vi "Query Relative Amplitude Limit Auto Enabled.vi"(8 "error in (no error)":errorcluster {"code" format="%.0x"}, 9 "RetValBufferSize":i32=2048, 11 "instrument handle":refnum<k15>) -> (0 "error out":errorcluster {"code" format="%.0x"}, 1 "RetValActualSize":i32, 2 "RetVal":u16[](array[numeric]), 3 "instrument handle out":refnum<k15>)   [LabVIEW 2021, in "Keysight XSAnVMA.lvlib"]
doc: "Gets state of relative power level limit at the stop frequency for the selected offset."
uses:
  <instrlib>/Keysight XSAnVMA/Keysight XSAnVMA.lvlib
  KtXSAnVMA_64.dll
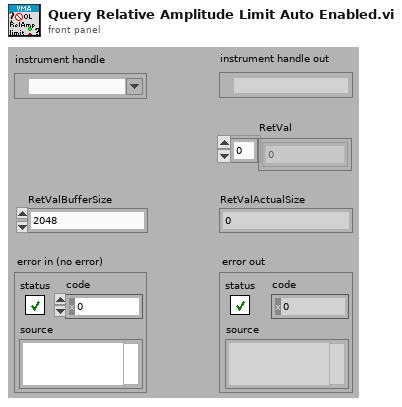
[diagram p1: front panel]
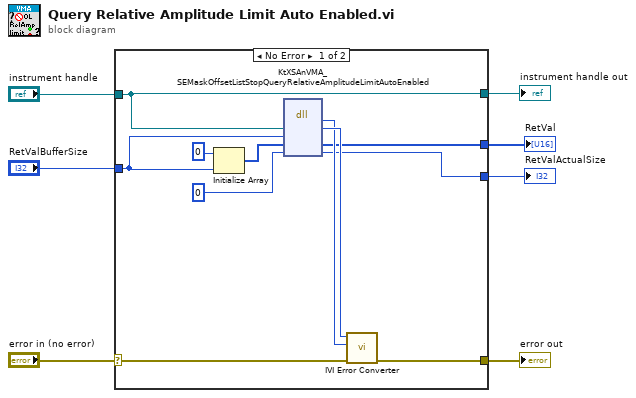
[diagram p0: block diagram]
diagram:
  n1 = case shown="No Error" "error in (no error)" {
    selector: "error in (no error)" -> [w16 w20]
    tunnel: [w15 w20] -> w7
    tunnel: "instrument handle" -> [w9 w19]
    tunnel: "RetValBufferSize" -> [w8 _]
    tunnel: [w12 _] -> w3
    tunnel: [w10 _] -> w2
    tunnel: [w9 w19] -> w1
    frame No Error {
      n2 = Initialize Array(u16 0 ("element"), w8) -> (w14:u16[])
      n3 = dll-call lib="KtXSAnVMA**.dll" fn="KtXSAnVMA_SEMaskOffsetListStopQueryRelativeAmplitudeLimitAutoEnabled"("Vi"=w9, "RetValBufferSize"=w8, "RetVal"=w14, "RetValActualSize"=0) -> (w17:i32, "Vi"=w18:u32, "RetVal"=w12:u16[], "RetValActualSize"=w10:i32)  [unwired: 4 in, 2 out]
      n4 = call <instrlib>:"IVI Error Converter.vi"("error in (no error)"=w16, "IVI error code (0)"=w17, "instrument handle"=w18) -> ("error out"=w15:errorcluster)  [unwired: 7 in, 1 out]
    }
    frame Error {
    }
  }
  "error out" <- w7
  "instrument handle out" <- w1
  "RetVal" <- w3
  "RetValActualSize" <- w2
